vi "Read WaitStarted.vi"(11 "SMO.DynamicLauncher in":refnum<class "SMO.DynamicLauncher.lvclass">) -> (2 "WaitStarted":bool, 3 "SMO.DynamicLauncher out":refnum<class "SMO.DynamicLauncher.lvclass">)   [LabVIEW 2013, in "SMO.DynamicLauncher.lvclass"]
uses:
  SMO.DynamicLauncher.lvclass
  SMO.DynamicLauncher.lvclass/SMO.DynamicLauncher.ctl
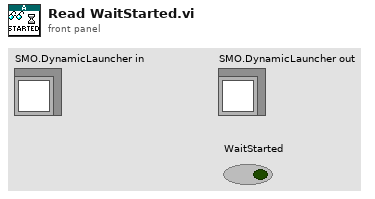
[diagram p1: front panel]
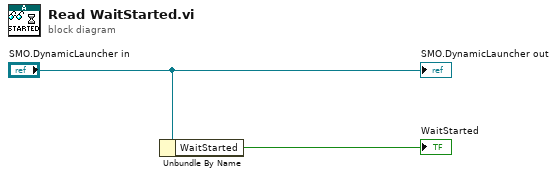
[diagram p0: block diagram]
diagram:
  n1 = Unbundle By Name("SMO.DynamicLauncher in") -> ("WaitStarted"=→"WaitStarted":bool)
  "SMO.DynamicLauncher out" <- "SMO.DynamicLauncher in"
